vi "Point Tool Histogram Result Values Compare.vi"(0 "Statistics":T2, 4 "Point Tool Histogram Limits":T1, 5 "error constant":errorcluster) -> (14 "Value":ext, 15 "Result":bool, 16 "Pass/Fail":bool, 17 "Area (pixels)":i32, 18 "Result(Area pixels)":bool, 19 "error constant":errorcluster)   [LabVIEW 2020]
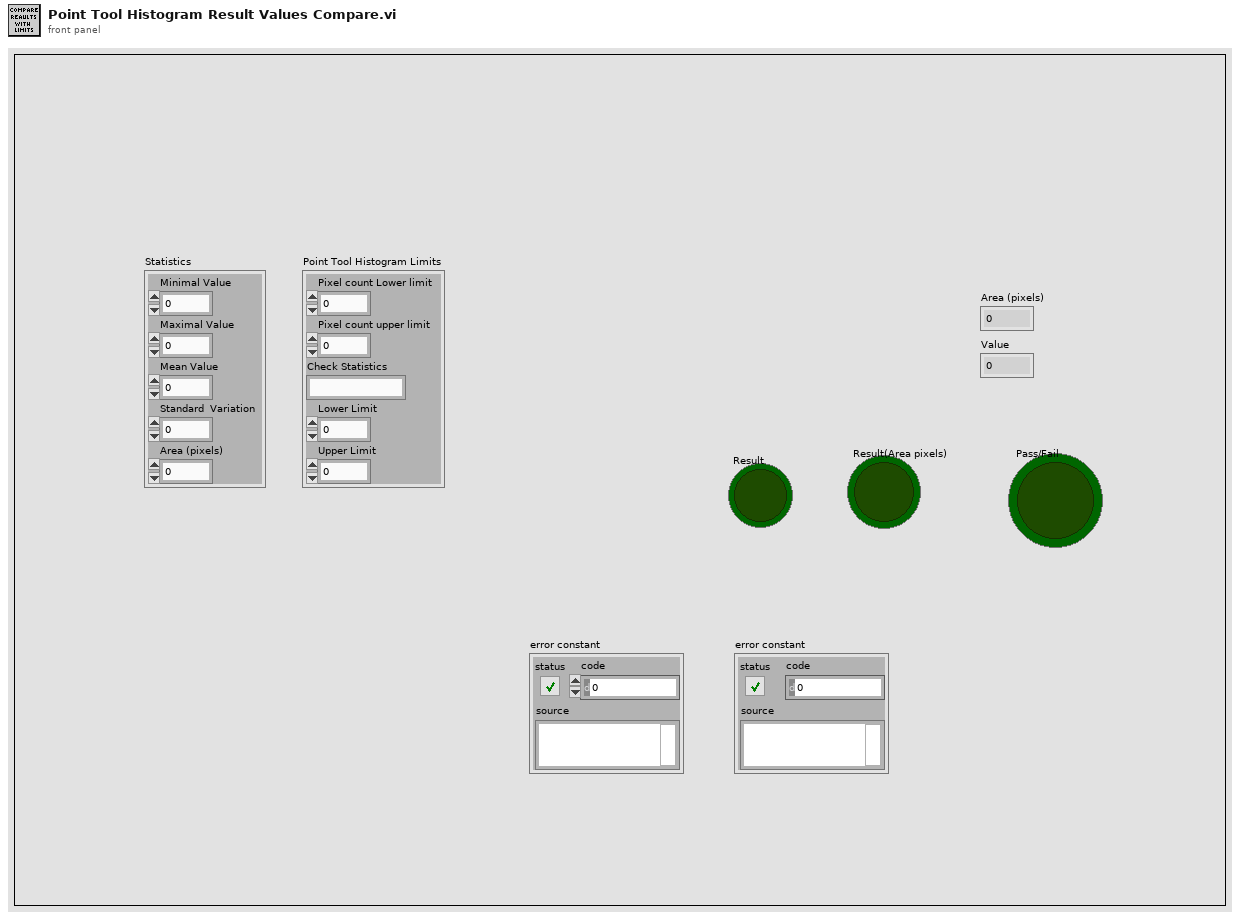
[diagram p1: front panel]
types:
  T1 = cluster{"Pixel count Lower limit":i32, "Pixel count upper limit":i32, "Check Statistics":string, "Lower Limit":i32, "Upper Limit":i32}
  T2 = cluster{"Minimal Value":sgl, "Maximal Value":sgl, "Mean Value":sgl, "Standard  Variation":sgl, "Area (pixels)":i32}
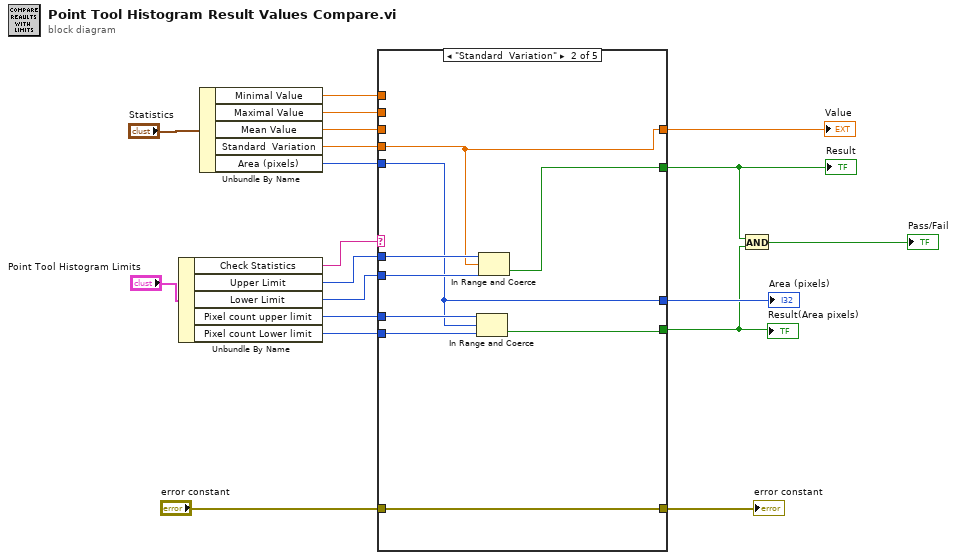
[diagram p0: block diagram]
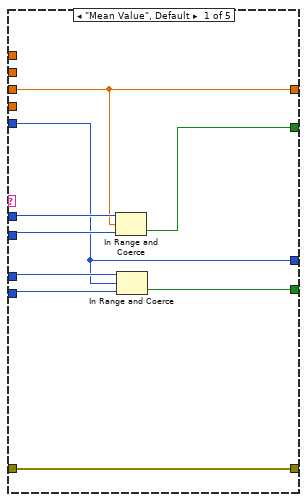
[diagram p2: hidden frame]
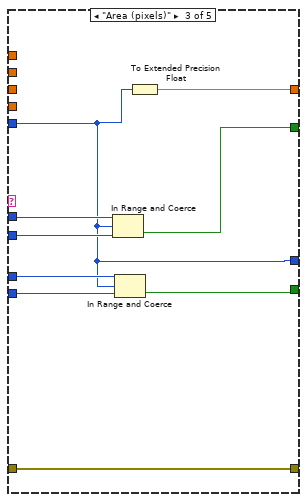
[diagram p3: hidden frame]
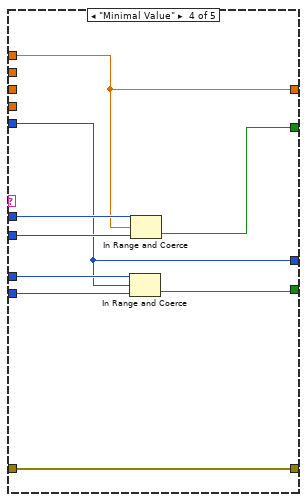
[diagram p4: hidden frame]
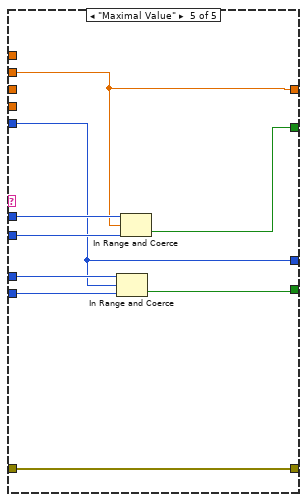
[diagram p5: hidden frame]
diagram:
  n1 = Unbundle By Name("Point Tool Histogram Limits") -> ("Check Statistics"=w10:string, "Upper Limit"=w18:i32, "Lower Limit"=w17:i32, "Pixel count upper limit"=w6:i32, "Pixel count Lower limit"=w5:i32)
  n2 = Unbundle By Name("Statistics") -> ("Minimal Value"=w15:sgl, "Maximal Value"=w14:sgl, "Mean Value"=w13:sgl, "Standard  Variation"=w12:sgl, "Area (pixels)"=w11:i32)
  n3 = case shown="\"Standard  Variation\"" w10 {
    tunnel: w15 -> [_ _ _ w52 _]
    tunnel: w14 -> [_ _ _ _ w61]
    tunnel: w13 -> [w25 _ _ _ _]
    tunnel: w12 -> [_ w34 _ _ _]
    tunnel: w11 -> [w21 w29 w38 w47 w56]
    tunnel: w18 -> [w28 w37 w46 w55 w64]
    tunnel: w17 -> [w27 w36 w45 w54 w63]
    tunnel: [w26 w35 w44 w53 w62] -> w2
    tunnel: [w25 w34 w43 w52 w61] -> w16
    tunnel: "error constant" -> [w24 w33 w42 w51 w60]
    tunnel: [w24 w33 w42 w51 w60] -> w8
    tunnel: w6 -> [w23 w31 w41 w50 w59]
    tunnel: w5 -> [w22 w32 w40 w49 w58]
    tunnel: [w21 w29 w38 w47 w56] -> w4
    tunnel: [w20 w30 w39 w48 w57] -> w3
    frame "Mean Value", Default {
      n4 = In Range and Coerce(upper limit=w28, x=w25, lower limit=w27) -> (In Range?=w26:bool)  [unwired: 1 out]
      n5 = In Range and Coerce(upper limit=w23, x=w21, lower limit=w22) -> (In Range?=w20:bool)  [unwired: 1 out]
    }
    frame "Standard  Variation" {
      n6 = In Range and Coerce(upper limit=w31, x=w29, lower limit=w32) -> (In Range?=w30:bool)  [unwired: 1 out]
      n7 = In Range and Coerce(upper limit=w37, x=w34, lower limit=w36) -> (In Range?=w35:bool)  [unwired: 1 out]
    }
    frame "Area (pixels)" {
      n8 = In Range and Coerce(upper limit=w46, x=w38, lower limit=w45) -> (In Range?=w44:bool)  [unwired: 1 out]
      n9 = In Range and Coerce(upper limit=w41, x=w38, lower limit=w40) -> (In Range?=w39:bool)  [unwired: 1 out]
      n10 = To Extended Precision Float(1:w38) -> (0:w43:ext)
    }
    frame "Minimal Value" {
      n11 = In Range and Coerce(upper limit=w50, x=w47, lower limit=w49) -> (In Range?=w48:bool)  [unwired: 1 out]
      n12 = In Range and Coerce(upper limit=w55, x=w52, lower limit=w54) -> (In Range?=w53:bool)  [unwired: 1 out]
    }
    frame "Maximal Value" {
      n13 = In Range and Coerce(upper limit=w59, x=w56, lower limit=w58) -> (In Range?=w57:bool)  [unwired: 1 out]
      n14 = In Range and Coerce(upper limit=w64, x=w61, lower limit=w63) -> (In Range?=w62:bool)  [unwired: 1 out]
    }
  }
  "Value" <- w16
  "Result" <- w2
  "error constant" <- w8
  "Area (pixels)" <- w4
  "Result(Area pixels)" <- w3
  n15 = And(x=w2, y=w3) -> (x .and. y?=→"Pass/Fail":bool)
